vi "Configure TX Port FIFO.vi"(8 "error in":errorcluster, 9 "FIFO Depth":u32, 10 "TX Port":T1 items=["Port 0", "Port 1", "Port 2", "Port 3"], 11 "Refnum in":refnum<k20>) -> (0 "error out":errorcluster, 1 "Actual Depth":u32, 3 "Refnum out":refnum<k20>)   [LabVIEW 2016, in "Aurora Stream (NI 6592R) (Host).lvlib"]
uses:
  Port.ctl
  Base Bitfile Reference.ctl
  <vilib>/rvi/interface/common/niFpgaWaitOnOcc.vi
  <vilib>/Utility/error.llb/Error Cluster From Error Code.vi
  <vilib>/rvi/interface/nirviMethod/nirviMethod.xnode
  Aurora Stream (NI 6592R) (Host).lvlib
  <vilib>/FPGAPlugInAG/Dynamic/niLvFpga_ConfigureFifo_Dynamic.vi
  <vilib>/rvi/errors/niLvFpgaMergeErrorWithErrorCode.vi
  <vilib>/FPGAPlugInAG/Dynamic/niLvFpga_StartFifo_Dynamic.vi
  <vilib>/FPGAPlugInAG/Dynamic/niLvFpga_StopFifo_Dynamic.vi
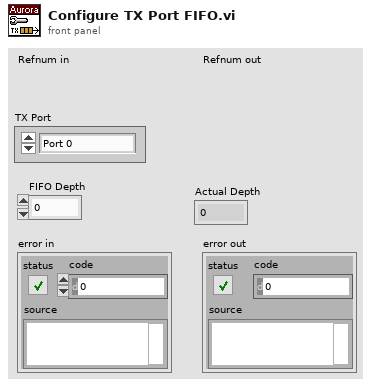
[diagram p1: front panel]
types:
  T1 = typedef "Aurora Stream (NI 6592R) (Host).lvlib/Port.ctl" = i32
  T2 = typedef "Aurora Stream (NI 6592R) (Host).lvlib/Base Bitfile Reference.ctl" = refnum<k20>
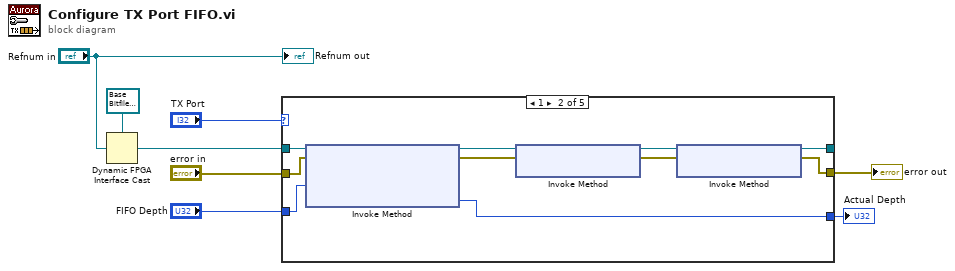
[diagram p0: block diagram]
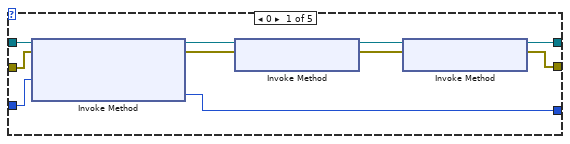
[diagram p2: hidden frame]
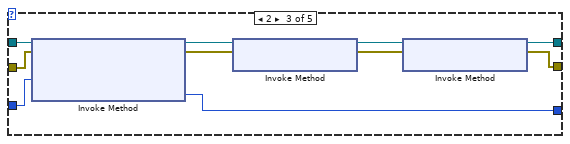
[diagram p3: hidden frame]
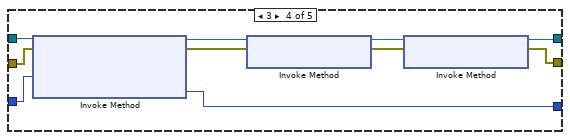
[diagram p4: hidden frame]
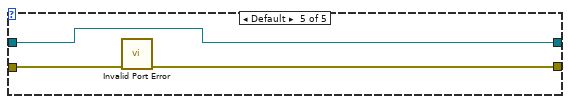
[diagram p5: hidden frame]
diagram:
  n1 = Dynamic FPGA Interface Cast(Session In=T2 refnum ("Aurora Sample Project"), Type="Refnum in") -> (Session Out=w3:T2)
  n2 = case shown="1" "TX Port" {
    tunnel: [w14 w25 w34 w44 w49] -> w6
    tunnel: w3 -> [w18 w28 w38 w48 w51]
    tunnel: "error in" -> [w17 w27 w37 w46 w50]
    tunnel: [w15 w26 w35 w45 w51] -> _
    tunnel: "FIFO Depth" -> [w16 w24 w36 w47 _]
    tunnel: [w13 w23 w33 w43 _] -> w1
    frame 0 {
      n3 = xnode "Invoke Method"("FPGA VI Reference In"=w18, "error in"=w17, "Requested Depth"=w16) -> ("FPGA VI Reference Out"=w12:T2, "error out"=w11:errorcluster, "Actual Depth"=w13:u32)
      n4 = xnode "Invoke Method"("FPGA VI Reference In"=w12, "error in"=w11) -> ("FPGA VI Reference Out"=w10:T2, "error out"=w9:errorcluster)
      n5 = xnode "Invoke Method"("FPGA VI Reference In"=w10, "error in"=w9) -> ("FPGA VI Reference Out"=w15:T2, "error out"=w14:errorcluster)
    }
    frame 1 {
      n6 = xnode "Invoke Method"("FPGA VI Reference In"=w28, "error in"=w27, "Requested Depth"=w24) -> ("FPGA VI Reference Out"=w22:T2, "error out"=w21:errorcluster, "Actual Depth"=w23:u32)
      n7 = xnode "Invoke Method"("FPGA VI Reference In"=w22, "error in"=w21) -> ("FPGA VI Reference Out"=w20:T2, "error out"=w19:errorcluster)
      n8 = xnode "Invoke Method"("FPGA VI Reference In"=w20, "error in"=w19) -> ("FPGA VI Reference Out"=w26:T2, "error out"=w25:errorcluster)
    }
    frame 2 {
      n9 = xnode "Invoke Method"("FPGA VI Reference In"=w38, "error in"=w37, "Requested Depth"=w36) -> ("FPGA VI Reference Out"=w32:T2, "error out"=w31:errorcluster, "Actual Depth"=w33:u32)
      n10 = xnode "Invoke Method"("FPGA VI Reference In"=w32, "error in"=w31) -> ("FPGA VI Reference Out"=w30:T2, "error out"=w29:errorcluster)
      n11 = xnode "Invoke Method"("FPGA VI Reference In"=w30, "error in"=w29) -> ("FPGA VI Reference Out"=w35:T2, "error out"=w34:errorcluster)
    }
    frame 3 {
      n12 = xnode "Invoke Method"("FPGA VI Reference In"=w48, "error in"=w46, "Requested Depth"=w47) -> ("FPGA VI Reference Out"=w42:T2, "error out"=w41:errorcluster, "Actual Depth"=w43:u32)
      n13 = xnode "Invoke Method"("FPGA VI Reference In"=w42, "error in"=w41) -> ("FPGA VI Reference Out"=w40:T2, "error out"=w39:errorcluster)
      n14 = xnode "Invoke Method"("FPGA VI Reference In"=w40, "error in"=w39) -> ("FPGA VI Reference Out"=w45:T2, "error out"=w44:errorcluster)
    }
    frame Default {
      n15 = call "Invalid Port Error.vi"("error in"=w50) -> ("error out"=w49:errorcluster)  [unwired: 14 in]
    }
  }
  "error out" <- w6
  "Actual Depth" <- w1
  "Refnum out" <- "Refnum in"
